vi "Pulse waveform generator.vi"(0 "Base waveform":waveform(dbl), 2 "Pulse Amplitude":dbl, 3 "Pulse Duration":dbl) -> (7 "Pulse waveform":waveform(dbl), 10 "real pulse duration":dbl)   [LabVIEW 2014]
uses:
  <vilib>/Waveform/WDTOps.llb/WDT Waveform Duration DBL.vi
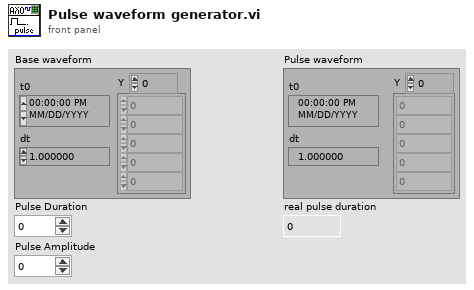
[diagram p1: front panel]
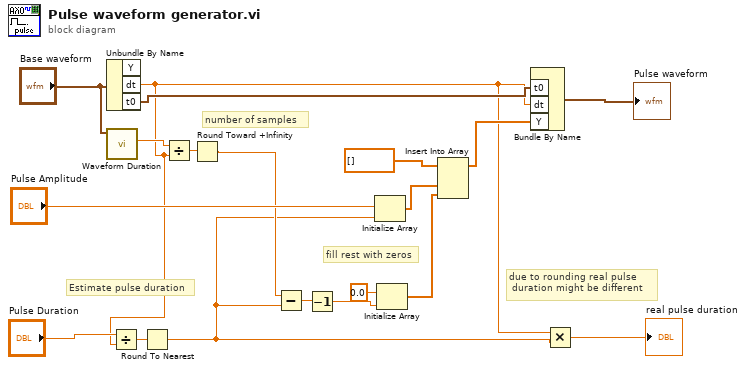
[diagram p0: block diagram]
diagram:
  # "due to rounding real pulse\n duration might be different"
  # "fill rest with zeros"
  # "Estimate pulse duration"
  # "number of samples"
  n1 = Unbundle By Name("Base waveform") -> ("dt"=w3:dbl, "t0"=w17:timestamp)  [unwired: 1 out]
  n2 = call-poly <vilib>:"Waveform Duration.vi"("waveform in"="Base waveform") -> ("duration"=w16:dbl)  [unwired: 8 in, 2 out]
  n3 = Divide(x="Pulse Duration", y=w3) -> (x/y=w12:dbl)
  n4 = Round To Nearest(number=w12) -> (nearest integer value=w2:dbl)
  n5 = Divide(x=w16, y=w3) -> (x/y=w8:dbl)
  n6 = Round Toward +Infinity(x=w8) -> (ceil(x): smallest int >= x=w7:dbl)
  n7 = Subtract(x=w7, y=w2) -> (x-y=w9:dbl)
  n8 = Decrement(x=w9) -> (x-1=w6:dbl)
  n9 = Initialize Array("Pulse Amplitude", w2) -> (w11:dbl[])
  n10 = Initialize Array(0.0 ("element"), w6) -> (w5:dbl[])
  n11 = Insert Into Array(array=dbl[] [], new element #1=w11, new element #2=w5) -> (w14:dbl[])  [unwired: 1 in]
  n12 = Bundle By Name("t0"=w17, "dt"=w3, "Y"=w14) -> (→"Pulse waveform":waveform(dbl))  [unwired: 1 in]
  n13 = Multiply(x=w3, y=w2) -> (x*y=→"real pulse duration":dbl)
